vi "getVXM.vi"(8 "error in (no error)":errorcluster, 9 "mmWave Axis Name":string="BS1", 11 "sub-systems in":refnum<class "sub-systems.lvclass">) -> (0 "error out":errorcluster, 1 "Axis (1..4)":T1=1 items=["X"=1, "Y"=2, "Z"=3, "T"=4], 2 "VXMx2 out":refnum<class "VXMx2.lvclass">, 3 "sub-systems out":refnum<class "sub-systems.lvclass">, 5 "Sub-syst number":i32)   [LabVIEW 2018, in "sub-systems.lvclass"]
doc: "return the VXM axis (X, Y, Z, T),\nthe VXM system containing the Axis\nand the sub-syst. number (1-3)"
uses:
  sub-systems.lvclass
  VSMx2/VXMx2.lvclass
  <instrlib>/Velmex VXM/Public/VXM Axis.ctl
  sub-systems.lvclass/sub-systems.ctl
  <instrlib>/Velmex VXM/Velmex VXM.lvlib
panel:
  # "This .ctl maybe shouldn't be \ncoupled up this high"
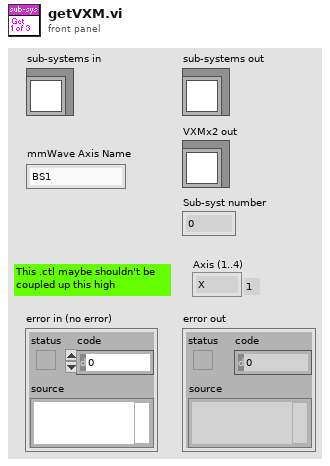
[diagram p1: front panel]
types:
  T1 = typedef "Velmex VXM.lvlib/VXM Axis.ctl" = u16
  T2 = cluster{"mmWaveName":string, "Sub-syst":i32, "Axis":string}[]
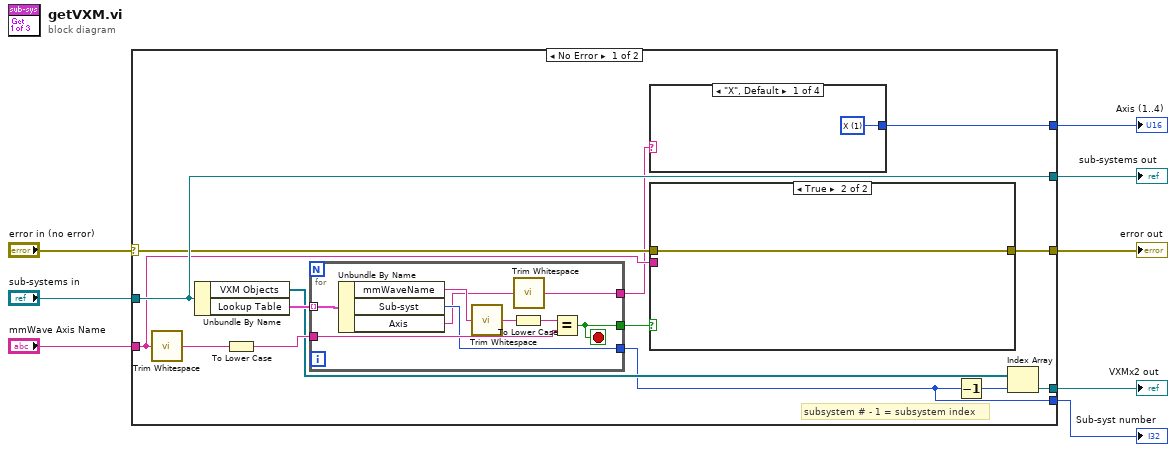
[diagram p0: block diagram]
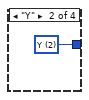
[diagram p2: hidden frame]
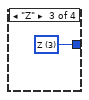
[diagram p3: hidden frame]
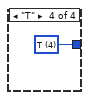
[diagram p4: hidden frame]
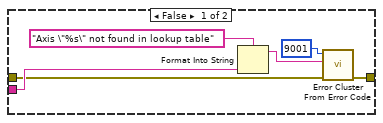
[diagram p5: hidden frame]
diagram:
  n1 = case shown="No Error" "error in (no error)" {
    selector: "error in (no error)" -> [w16 w44]
    tunnel: [w15 w44] -> w7
    tunnel: [w22 w43] -> w5
    tunnel: "sub-systems in" -> [w22 w43]
    tunnel: "mmWave Axis Name" -> [w17 _]
    tunnel: [w13 _] -> w3
    tunnel: [w9 _] -> w2
    tunnel: [w11 _] -> w1
    frame No Error {
      # "subsystem # - 1 = subsystem index"
      n2 = call <vilib>:"Trim Whitespace.vi"("string"=w17) -> ("trimmed string"=w19:string)  [unwired: 1 in]
      n3 = Unbundle By Name(w22) -> ("VXM Objects"=w18:refnum<class "VXMx2.lvclass">[], "Lookup Table"=w21:T2)
      n4 = To Lower Case(string=w19) -> (all lower case string=w20:string)
      n5 = for {
        tunnel: w21 -> [w42] mode=indexing
        tunnel: w20 -> [w38]
        tunnel: [w37] -> w14
        tunnel: [w36] -> w9
        tunnel: [w34] -> w12
        stop <- w37 stop-if-true
        n6 = Unbundle By Name(w42) -> ("mmWaveName"=w41:string, "Sub-syst"=w36:i32, "Axis"=w35:string)
        n7 = call <vilib>:"Trim Whitespace.vi"("string"=w41) -> ("trimmed string"=w40:string)  [unwired: 1 in]
        n8 = To Lower Case(string=w40) -> (all lower case string=w39:string)
        n9 = call <vilib>:"Trim Whitespace.vi"("string"=w35) -> ("trimmed string"=w34:string)  [unwired: 1 in]
        n10 = Equal?(x=w39, y=w38) -> (x = y?=w37:bool)
      }
      n11 = case shown="\"X\", Default" w12 {
        tunnel: [w23 w24 w25 w26] -> w11
        frame "X", Default {
          w23 = T1 1 items=["X"=1, "Y"=2, "Z"=3, "T"=4] ("Axis (1..4)")
        }
        frame "Y" {
          w24 = T1 2 items=["X"=1, "Y"=2, "Z"=3, "T"=4] ("Axis (1..4)")
        }
        frame "Z" {
          w25 = T1 3 items=["X"=1, "Y"=2, "Z"=3, "T"=4] ("Axis (1..4)")
        }
        frame "T" {
          w26 = T1 4 items=["X"=1, "Y"=2, "Z"=3, "T"=4] ("Axis (1..4)")
        }
      }
      n12 = case shown="True" w14 {
        tunnel: w17 -> [w29 _]
        tunnel: w16 -> [w28 w33]
        tunnel: [w27 w33] -> w15
        frame False {
          n13 = Format Into String(format string="Axis \"%s\" not found in lookup table", w29) -> (resulting string=w30:string)  [unwired: 2 in, 1 out]
          n14 = call <vilib>:"Error Cluster From Error Code.vi"("error in (no error)"=w28, "error message (\"\")"=w30, "error code (0)"=9001) -> ("error out"=w27:errorcluster)  [unwired: 6 in]
        }
        frame True {
        }
      }
      n15 = Decrement(x=w9) -> (x-1=w10:i32)
      n16 = Index Array(array=w18, index=w10) -> (element=w13:refnum<class "VXMx2.lvclass">)
    }
    frame Error {
    }
  }
  "error out" <- w7
  "sub-systems out" <- w5
  "VXMx2 out" <- w3
  "Sub-syst number" <- w2
  "Axis (1..4)" <- w1
